vi "RT_Proof of Concept.vi"() -> ()   [LabVIEW 2010]
uses:
  <vilib>/Platform/TimedLoop/XDataNode/XDataNode.xnode
  <vilib>/Platform/TimedLoop/XDataNode/timing_clust.ctl
  <vilib>/Platform/TimedLoop/XDataNode/nitl_modes.ctl
  <vilib>/Platform/TimedLoop/XDataNode/wakeup.ctl
  <vilib>/Utility/error.llb/DialogType.ctl
  <vilib>/Pansino Software/LabVIEW Architecture/PSARC_Queue Management.llb/PSARC_Queue Insert Element.vi
  <vilib>/Platform/TimedLoop/XDataNode/XDNodeRunTimeDep.lvlib
panel:
  out "x+1":i32
  out "Error Report":string
  in  "Exit":bool
  in  "OK":bool
  out "Current State":string
  in  "Temp Variable":cluster{"Error":errorcluster, "Exit":bool}
  # "————————————————\nYou could add your temporary variables\nhere.\nThis Control should be saved as a\nvi in your project folder,The proposed vi's block diagram is shown in the picture\n\n\n\n\n\n\n\n————————————————"
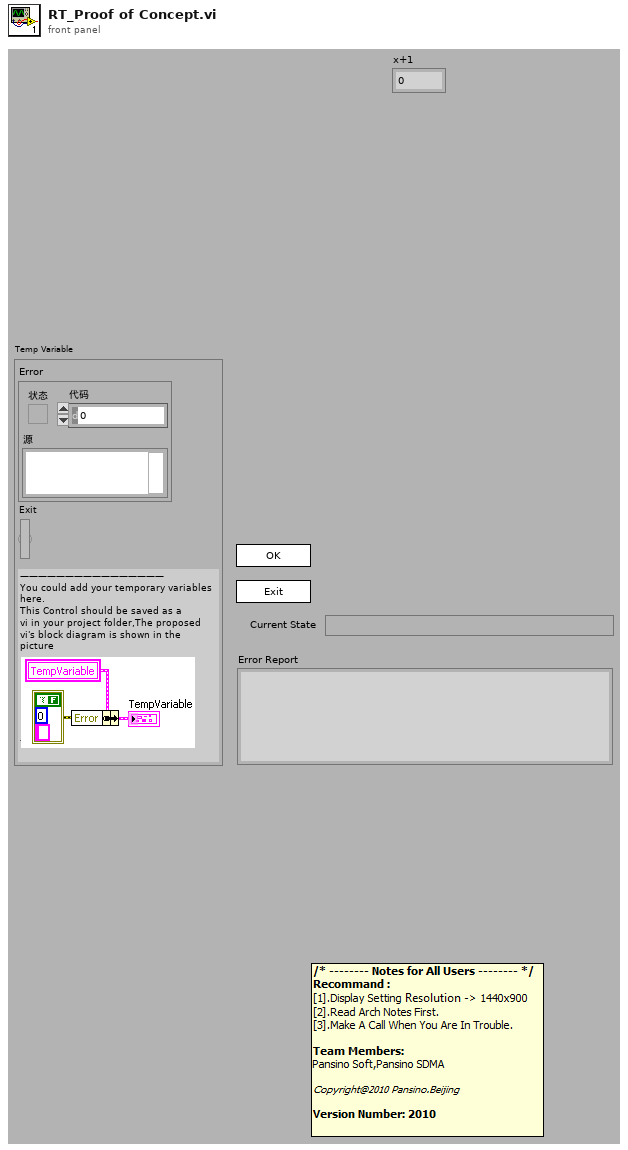
[diagram p1: front panel]
types:
  T1 = typedef "XDNodeRunTimeDep.lvlib/timing_clust.ctl" = cluster{"Expected End [f-1]":u64, "Actual End [f-1]":u64, "Finished Late? [f-1]":bool, "Expected End [i-1]":u64, "Actual End [i-1]":u64, "Finished Late? [i-1]":bool, "Expected Start [i]":u64, "Actual Start [i]":u64, "Expected Start [f]":u64, "Actual Start [f]":u64, "Source Name":string, "Structure Name":string, "Period":i64, "Deadline":i64, "Offset":i64, "Start":i64, "Priority":i32, "Timeout":i32, "Mode":T2, "Wakeup Reason":T3, "Error":errorcluster, "Source Type":string, "Secondary Source Type":string, "Global End Time":u64, "Global Start Time":u64, "Frame Duration":u64, "Iteration Duration":u64, "Assigned CPU":i32, "I/O Scan Engine Mode":u32}
  T2 = typedef "XDNodeRunTimeDep.lvlib/nitl_modes.ctl" = enum32{"No Change", "Process missed periods, maintain original phase", "Discard missed periods, maintain original phase", "Process missed periods, ignore original phase", "Discard missed periods, ignore original phase"}
  T3 = typedef "XDNodeRunTimeDep.lvlib/wakeup.ctl" = enum32{"Normal", "Aborted", "Asynchronous wakeup", "Timing source error", "Timed loop error", "Timeout"}
  T4 = typedef "DialogType.ctl" = u16
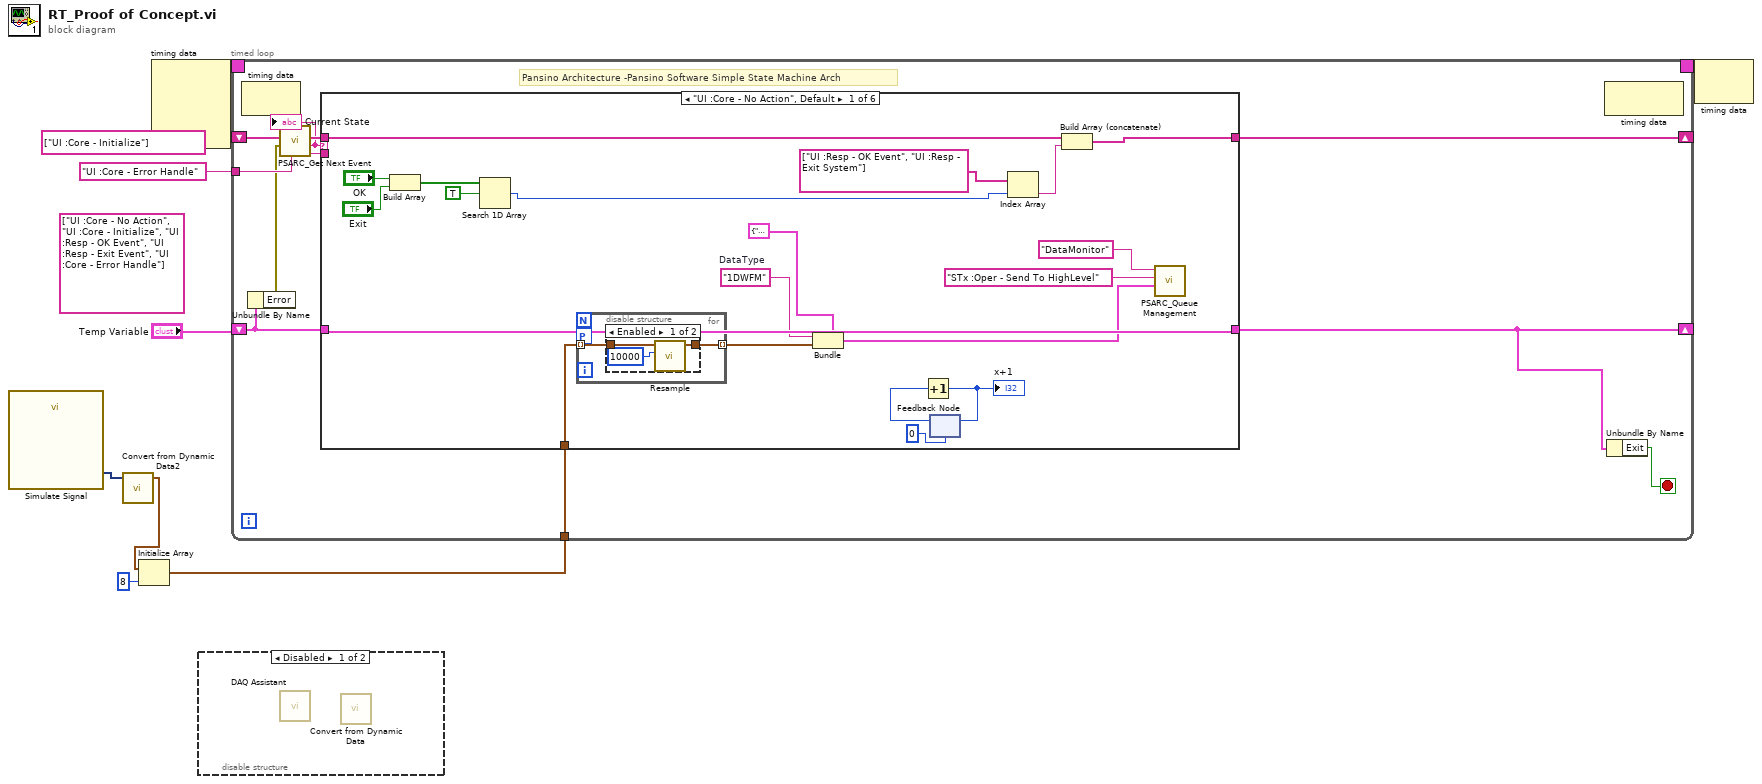
[diagram p0: block diagram]
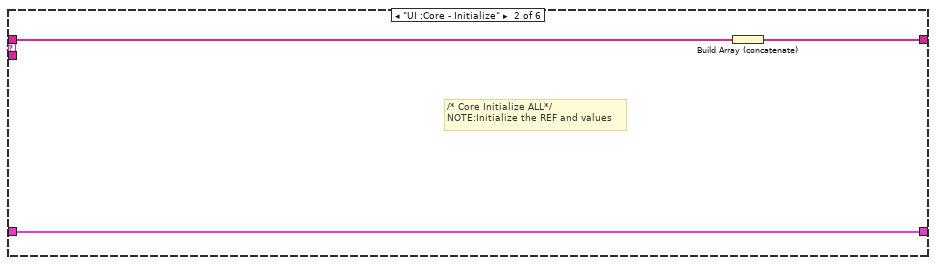
[diagram p3: hidden frame]
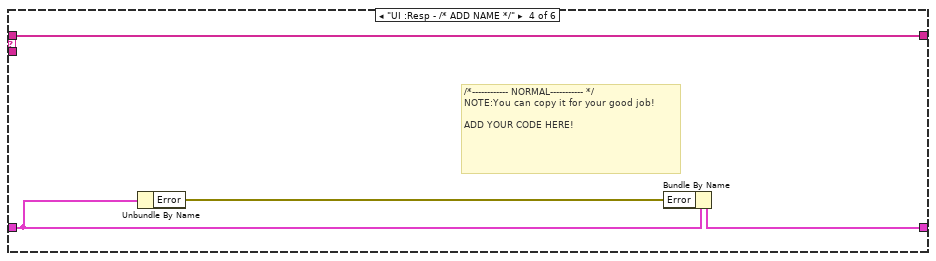
[diagram p5: hidden frame]
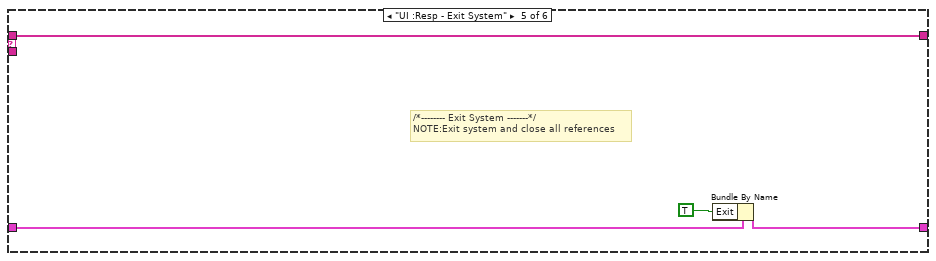
[diagram p6: hidden frame]
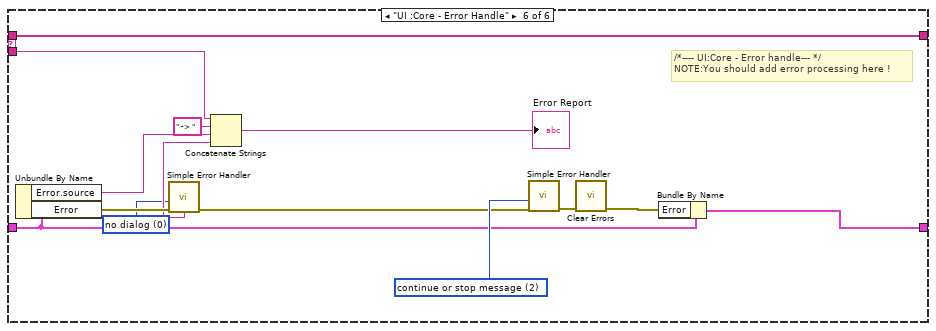
[diagram p7: hidden frame]
diagram:
  (unwired) string[] ["UI :Core - No Action", "UI :Core - Initialize", "UI :Resp - OK Event", "UI :Resp - Exit Event", "UI :Core - Error Handle"]
  n1 = call "Simulate Signal"() -> ("Sine"=w6:dynamicdata)  [unwired: 14 in, 1 out]
  n2 = call "Convert from Dynamic Data2"("Dynamic Data Type"=w6) -> ("Waveform"=w5:waveform(dbl))  [unwired: 3 in]
  n3 = Initialize Array(w5, 8 ("dimension size")) -> (w3:waveform(dbl)[])
  n4 = node-c288() -> (w2:T1)  [unwired: 4 in]
  n5 = disable-structure shown="Disabled" {
    frame Disabled {
      n6 = call "DAQ Assistant"() -> ()  [unwired: 16 in, 4 out]
      n7 = call "Convert from Dynamic Data"() -> ()  [unwired: 4 in, 1 out]
    }
    frame Enabled {
    }
  }
  n8 = timed-loop {
    tunnel: "UI :Core - Error Handle" ("Error Handle") -> [w19]
    shift-right: [w17] -> _
    shift-left: string[] ["UI :Core - Initialize"] -> [w20]
    shift-right: [w14] -> _
    shift-left: "Temp Variable" -> [w16]
    tunnel: w3 -> [w10]
    timing: w2 -> [_]
    timing-out: [_] -> w1
    stop <- w13 stop-if-true
    # "Pansino Architecture -Pansino Software Simple State Machine Arch"
    n9 = node-c288() -> ()  [unwired: 1 in, 1 out]
    n10 = Unbundle By Name(w16) -> ("Error"=w15:errorcluster)
    n11 = call <vilib>:"PSARC_Get Next Event.vi"("Error Handle"=w19, "error in (no error)"=w15, "event queue in"=w20) -> ("prev event"=w11:string, "next event"=w12:string, "event queue out"=w18:string[])  [unwired: 3 in]
    "Current State" <- w12
    n12 = case shown="\"UI :Core - No Action\", Default" w12 {
      tunnel: w18 -> [w35 w50 w52 w56 w60 w74]
      tunnel: [w34 w48 w52 w56 w60 w74] -> w17
      tunnel: w16 -> [w42 w49 w51 w55 w59 w71]
      tunnel: [w42 w49 w51 w54 w58 w70] -> w14
      tunnel: w11 -> [_ _ _ _ _ w63]
      tunnel: w10 -> [w23 _ _ _ _ _]
      frame "UI :Core - No Action", Default {
        w29 = "1DWFM"  # DataType
        n13 = Build Array("OK", "Exit") -> (w39:bool[])
        n14 = Search 1D Array(1D array=w39, element=TRUE ("元素")) -> (index of element=w36:i32)  [unwired: 1 in]
        n15 = for {
          tunnel: w23 -> [w44] mode=indexing
          tunnel: [w43] -> w24 mode=indexing
          workers-P: _ -> [_]
          n16 = disable-structure shown="Enabled" {
            disable-tunnel: w44 -> [w47 _]
            disable-tunnel: [w46 _] -> w43
            frame Enabled {
              n17 = call "Resample.vi"("Divide by"=10000, "Waveform"=w47) -> ("output waveform"=w46:waveform(dbl))  [unwired: 9 in]
            }
            frame Disabled {
            }
          }
        }
        n18 = Bundle(cluster=cluster{"DataType":string, "Data":variant} {"DataType"="", "Data"=variant}, "DataType"=w29, "Data"=w24) -> (w30:cluster{"DataType":string, "Data":variant})
        n19 = feedback #1(0) -> (w27:i32)
        n20 = Increment(x=w27) -> (x+1=w25:i32)
        "x+1" <- w25
        n21 = feedback-in #1(w25) -> ()
        n22 = Index Array(array=string[] ["UI :Resp - OK Event", "UI :Resp - Exit System"], index=w36) -> (element=w33:string)
        n23 = Build Array (concatenate)(w35, w33) -> (w34:string[])
        n24 = call-poly <vilib>:"PSARC_Queue Management.vi"("Data"=w30, "Event"="STx :Oper - Send To HighLevel", "Queue Name(unamed)"="DataMonitor") -> ()  [unwired: 7 in, 2 out]
      }
      frame "UI :Core - Initialize" {
        # "/* Core Initialize ALL*/\nNOTE:Initialize the REF and values"
        n25 = Build Array (concatenate)(w50) -> (w48:string[])
      }
      frame "UI :Resp - OK Event" {
      }
      frame "UI :Resp - /* ADD NAME */" {
        # "/*------------ NORMAL----------- */\nNOTE:You can copy it for your good job!\n\nADD YOUR CODE HERE!"
        n26 = Unbundle By Name(w55) -> ("Error"=w53:errorcluster)
        n27 = Bundle By Name(cluster=w55, "Error"=w53) -> (w54:cluster{"Error":errorcluster, "Exit":bool})
      }
      frame "UI :Resp - Exit System" {
        # "/*-------- Exit System -------*/\nNOTE:Exit system and close all references"
        n28 = Bundle By Name(cluster=w59, "Exit"=TRUE) -> (w58:cluster{"Error":errorcluster, "Exit":bool})
      }
      frame "UI :Core - Error Handle" {
        w61 = T4 0 items=["no dialog", "OK message", "continue or stop message", "OK message + warnings", "continue/stop + warnings"] ("type of dialog (OK msg:1)")
        w73 = T4 2 items=["no dialog", "OK message", "continue or stop message", "OK message + warnings", "continue/stop + warnings"] ("type of dialog (OK msg:1)")
        # "/*---- UI:Core - Error handle--- */\nNOTE:You should add error processing here !"
        n29 = Unbundle By Name(w71) -> ("Error.source"=w67:string, "Error"=w68:errorcluster)
        n30 = call <vilib>:"Simple Error Handler.vi"("type of dialog (OK msg:1)"=w61, "error in (no error)"=w68) -> ("error out"=w66:errorcluster, "message"=w65:string)  [unwired: 3 in, 3 out]
        n31 = Concatenate Strings(w63, " -> " ("字符串"), w67, w65) -> (→"Error Report":string)
        n32 = call <vilib>:"Simple Error Handler.vi"("type of dialog (OK msg:1)"=w73, "error in (no error)"=w66) -> ("error out"=w72:errorcluster)  [unwired: 3 in, 4 out]
        n33 = call <vilib>:"Clear Errors.vi"("error in (no error)"=w72) -> ("error out"=w69:errorcluster)  [unwired: 6 in]
        n34 = Bundle By Name(cluster=w71, "Error"=w69) -> (w70:cluster{"Error":errorcluster, "Exit":bool})
      }
    }
    n35 = node-c288() -> ()  [unwired: 1 in, 1 out]
    n36 = Unbundle By Name(w14) -> ("Exit"=w13:bool)
  }
  n37 = node-c288(w1) -> ()  [unwired: 1 out]
